vi "Convert_InstrumentReferenceArray_2_ChannelReferenceArray.vi"(2 "error in (no error)":errorcluster, 3 "DCPowerInformationClusterArray_Input":T2(array[cluster])) -> (0 "error out":errorcluster, 1 "DCPowerInformation_byChannel":T1(array[cluster]))   [LabVIEW 2019]
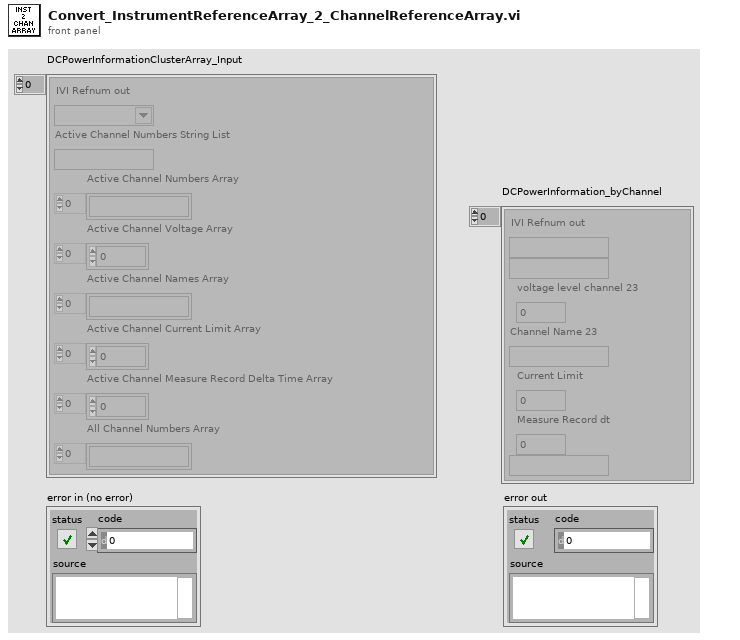
[diagram p1: front panel]
types:
  T1 = cluster{"IVI Refnum out":refnum<k15>, string, "voltage level channel 23":dbl, "Channel Name 23":string, "Current Limit":dbl, "Measure Record dt":dbl, string}[]
  T2 = cluster{"IVI Refnum out":refnum<k15>, "Active Channel Numbers String List":string, "Active Channel Numbers Array":string[], "Active Channel Voltage Array":dbl[], "Active Channel Names Array":string[], "Active Channel Current Limit Array":dbl[], "Active Channel Measure Record Delta Time Array":dbl[], "All Channel Numbers Array":string[]}[]
  T3 = cluster{"IVI Refnum out":refnum<k15>, string, "voltage level channel 23":dbl, "Channel Name 23":string, "Current Limit":dbl, "Measure Record dt":dbl, string}
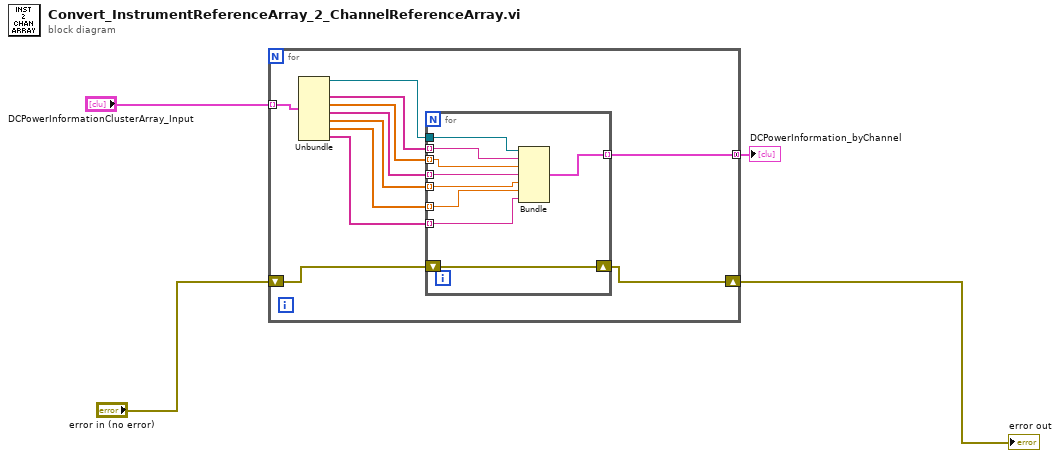
[diagram p0: block diagram]
diagram:
  n1 = for {
    tunnel: "DCPowerInformationClusterArray_Input" -> [w15] mode=indexing
    tunnel: [w12] -> w1 mode=concatenating
    shift-right: [w11] -> w4
    shift-left: "error in (no error)" -> [w10]
    n2 = Unbundle(w15) -> ("IVI Refnum out"=w14:refnum<k15>, "Active Channel Numbers Array"=w13:string[], "Active Channel Voltage Array"=w9:dbl[], "Active Channel Names Array"=w8:string[], "Active Channel Current Limit Array"=w7:dbl[], "Active Channel Measure Record Delta Time Array"=w6:dbl[], "All Channel Numbers Array"=w5:string[])  [unwired: 1 out]
    n3 = for {
      tunnel: w14 -> [w24]
      tunnel: w13 -> [w21] mode=indexing
      tunnel: [w23] -> w12 mode=indexing
      shift-right: [w22] -> w11
      shift-left: w10 -> [w22]
      tunnel: w9 -> [w20] mode=indexing
      tunnel: w8 -> [w19] mode=indexing
      tunnel: w7 -> [w18] mode=indexing
      tunnel: w6 -> [w17] mode=indexing
      tunnel: w5 -> [w16] mode=indexing
      n4 = Bundle("IVI Refnum out"=w24, w21, "voltage level channel 23"=w20, "Channel Name 23"=w19, "Current Limit"=w18, "Measure Record dt"=w17, w16) -> (w23:T3)  [unwired: 1 in]
    }
  }
  "error out" <- w4
  "DCPowerInformation_byChannel" <- w1
